vi "ServerRedo.vi"() -> ()   [LabVIEW 2021]
panel:
  in  "stop":bool
  in  "Tamper":cluster{u32, u32}[](array[cluster])
  in  "Alarm":cluster{u32, u32}[](array[cluster])
  in  "Bypass":cluster{u32, u32}[](array[cluster])
  in  "Normal":cluster{u32, u32}[](array[cluster])
  out "Zone 6":bool
  out "Zone 5":bool
  out "Zone 4":bool
  out "Zone 3":bool
  out "Zone 2":bool
  out "Zone 1":bool
  # "Green = Normal\nRed = Alarm\nOrange = Tamper\nBlue = Bypass"
  # "Zone Status Indicators"
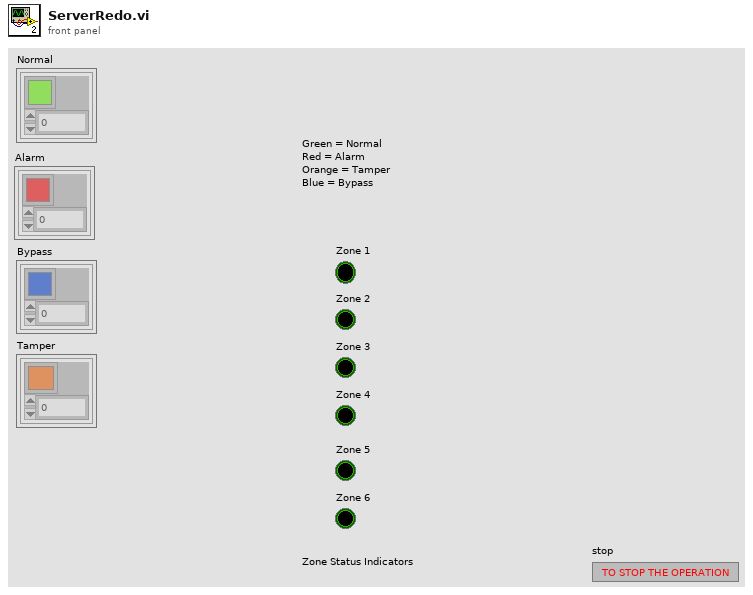
[diagram p1: front panel]
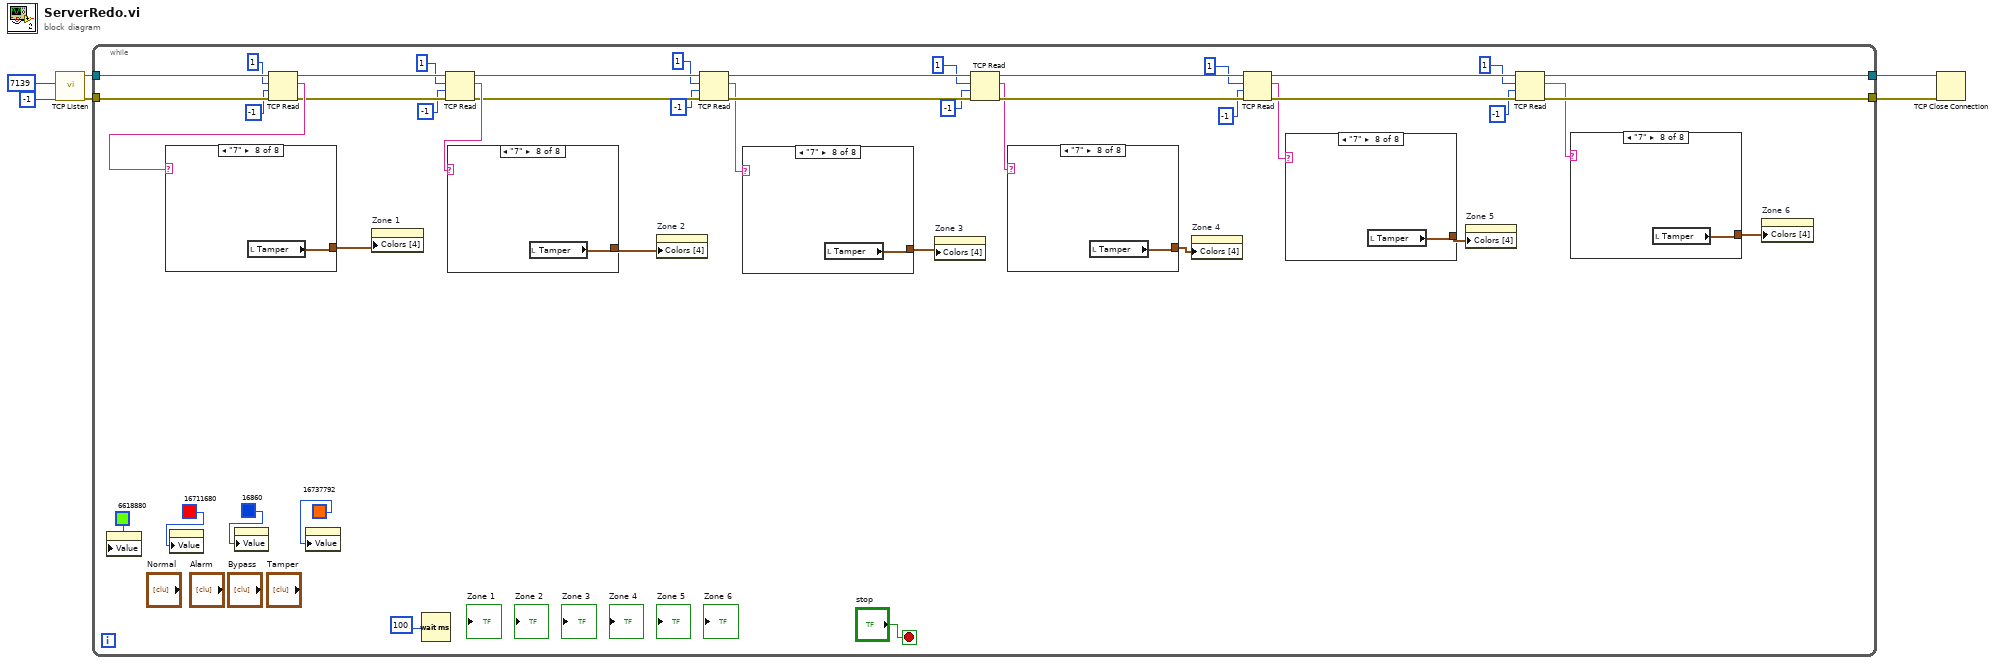
[diagram p0: block diagram]
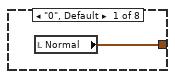
[diagram p2: hidden frame]
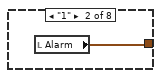
[diagram p3: hidden frame]
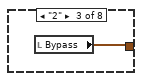
[diagram p4: hidden frame]
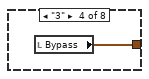
[diagram p5: hidden frame]
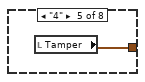
[diagram p6: hidden frame]
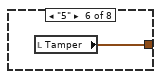
[diagram p7: hidden frame]
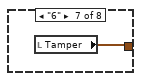
[diagram p8: hidden frame]
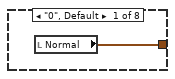
[diagram p9: hidden frame]
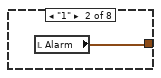
[diagram p10: hidden frame]
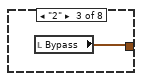
[diagram p11: hidden frame]
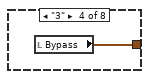
[diagram p12: hidden frame]
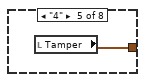
[diagram p13: hidden frame]
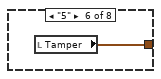
[diagram p14: hidden frame]
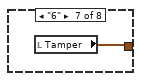
[diagram p15: hidden frame]
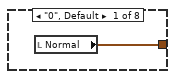
[diagram p16: hidden frame]
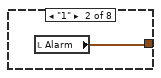
[diagram p17: hidden frame]
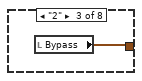
[diagram p18: hidden frame]
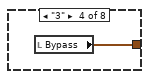
[diagram p19: hidden frame]
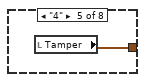
[diagram p20: hidden frame]
diagram:
  n1 = call <vilib>:"TCP Listen.vi"("timeout ms (wait forever: -1)"=-1, "port"=u16 7139) -> ("error out"=w2:errorcluster, "connection ID"=w4:refnum<k5>)  [unwired: 5 in, 3 out]
  n2 = while {
    tunnel: w4 -> [w50]
    tunnel: [w27] -> w3
    tunnel: w2 -> [w49]
    tunnel: [w23] -> w1
    stop <- "stop" stop-if-true
    n3 = property class="ColBox"("Value"=u32 6618880) -> ()  [unwired: 2 in, 2 out]
    n4 = property class="ColBox"("Value"=u32 16711680) -> ()  [unwired: 2 in, 2 out]
    n5 = property class="ColBox"("Value"=u32 16860) -> ()  [unwired: 2 in, 2 out]
    n6 = TCP Read(connection ID=w50, bytes to read=1, error in (no error)=w49, 9:-1 ("timeout ms (25000)")) -> (connection ID out=w38:refnum<k5>, data out=w46:string, error out=w37:errorcluster)  [unwired: 1 in]
    n7 = case shown="\"7\"" w46 {
      tunnel: [w91 w92 w93 w94 w95 w96 w97 w98] -> w45
      frame "0", Default {
        n8 = local read "Normal"() -> (w91:cluster{u32, u32}[])
      }
      frame "1" {
        n9 = local read "Alarm"() -> (w92:cluster{u32, u32}[])
      }
      frame "2" {
        n10 = local read "Bypass"() -> (w93:cluster{u32, u32}[])
      }
      frame "3" {
        n11 = local read "Bypass"() -> (w94:cluster{u32, u32}[])
      }
      frame "4" {
        n12 = local read "Tamper"() -> (w95:cluster{u32, u32}[])
      }
      frame "5" {
        n13 = local read "Tamper"() -> (w96:cluster{u32, u32}[])
      }
      frame "6" {
        n14 = local read "Tamper"() -> (w97:cluster{u32, u32}[])
      }
      frame "7" {
        n15 = local read "Tamper"() -> (w98:cluster{u32, u32}[])
      }
    }
    n16 = property class="ColBox"("Value"=u32 16737792) -> ()  [unwired: 2 in, 2 out]
    n17 = property on="Zone 1" class="Bool (strict)"("Colors [4]"=w45) -> ()  [unwired: 2 in, 2 out]
    n18 = Wait (ms)(milliseconds to wait=100) -> ()  [unwired: 1 out]
    n19 = TCP Read(connection ID=w38, bytes to read=1, error in (no error)=w37, 9:-1 ("timeout ms (25000)")) -> (connection ID out=w32:refnum<k5>, data out=w35:string, error out=w28:errorcluster)  [unwired: 1 in]
    n20 = case shown="\"7\"" w35 {
      tunnel: [w83 w84 w85 w86 w87 w88 w89 w90] -> w36
      frame "0", Default {
        n21 = local read "Normal"() -> (w83:cluster{u32, u32}[])
      }
      frame "1" {
        n22 = local read "Alarm"() -> (w84:cluster{u32, u32}[])
      }
      frame "2" {
        n23 = local read "Bypass"() -> (w85:cluster{u32, u32}[])
      }
      frame "3" {
        n24 = local read "Bypass"() -> (w86:cluster{u32, u32}[])
      }
      frame "4" {
        n25 = local read "Tamper"() -> (w87:cluster{u32, u32}[])
      }
      frame "5" {
        n26 = local read "Tamper"() -> (w88:cluster{u32, u32}[])
      }
      frame "6" {
        n27 = local read "Tamper"() -> (w89:cluster{u32, u32}[])
      }
      frame "7" {
        n28 = local read "Tamper"() -> (w90:cluster{u32, u32}[])
      }
    }
    n29 = property on="Zone 2" class="Bool (strict)"("Colors [4]"=w36) -> ()  [unwired: 2 in, 2 out]
    n30 = TCP Read(connection ID=w32, bytes to read=1, error in (no error)=w28, 9:-1 ("timeout ms (25000)")) -> (connection ID out=w31:refnum<k5>, data out=w13:string, error out=w26:errorcluster)  [unwired: 1 in]
    n31 = case shown="\"7\"" w13 {
      tunnel: [w75 w76 w77 w78 w79 w80 w81 w82] -> w14
      frame "0", Default {
        n32 = local read "Normal"() -> (w75:cluster{u32, u32}[])
      }
      frame "1" {
        n33 = local read "Alarm"() -> (w76:cluster{u32, u32}[])
      }
      frame "2" {
        n34 = local read "Bypass"() -> (w77:cluster{u32, u32}[])
      }
      frame "3" {
        n35 = local read "Bypass"() -> (w78:cluster{u32, u32}[])
      }
      frame "4" {
        n36 = local read "Tamper"() -> (w79:cluster{u32, u32}[])
      }
      frame "5" {
        n37 = local read "Tamper"() -> (w80:cluster{u32, u32}[])
      }
      frame "6" {
        n38 = local read "Tamper"() -> (w81:cluster{u32, u32}[])
      }
      frame "7" {
        n39 = local read "Tamper"() -> (w82:cluster{u32, u32}[])
      }
    }
    n40 = property on="Zone 3" class="Bool (strict)"("Colors [4]"=w14) -> ()  [unwired: 2 in, 2 out]
    n41 = TCP Read(connection ID=w31, bytes to read=1, error in (no error)=w26, 9:-1 ("timeout ms (25000)")) -> (connection ID out=w30:refnum<k5>, data out=w7:string, error out=w25:errorcluster)  [unwired: 1 in]
    n42 = case shown="\"7\"" w7 {
      tunnel: [w67 w68 w69 w70 w71 w72 w73 w74] -> w12
      frame "0", Default {
        n43 = local read "Normal"() -> (w67:cluster{u32, u32}[])
      }
      frame "1" {
        n44 = local read "Alarm"() -> (w68:cluster{u32, u32}[])
      }
      frame "2" {
        n45 = local read "Bypass"() -> (w69:cluster{u32, u32}[])
      }
      frame "3" {
        n46 = local read "Bypass"() -> (w70:cluster{u32, u32}[])
      }
      frame "4" {
        n47 = local read "Tamper"() -> (w71:cluster{u32, u32}[])
      }
      frame "5" {
        n48 = local read "Tamper"() -> (w72:cluster{u32, u32}[])
      }
      frame "6" {
        n49 = local read "Tamper"() -> (w73:cluster{u32, u32}[])
      }
      frame "7" {
        n50 = local read "Tamper"() -> (w74:cluster{u32, u32}[])
      }
    }
    n51 = property on="Zone 4" class="Bool (strict)"("Colors [4]"=w12) -> ()  [unwired: 2 in, 2 out]
    n52 = TCP Read(connection ID=w30, bytes to read=1, error in (no error)=w25, 9:-1 ("timeout ms (25000)")) -> (connection ID out=w29:refnum<k5>, data out=w8:string, error out=w24:errorcluster)  [unwired: 1 in]
    n53 = case shown="\"7\"" w8 {
      tunnel: [w59 w60 w61 w62 w63 w64 w65 w66] -> w11
      frame "0", Default {
        n54 = local read "Normal"() -> (w59:cluster{u32, u32}[])
      }
      frame "1" {
        n55 = local read "Alarm"() -> (w60:cluster{u32, u32}[])
      }
      frame "2" {
        n56 = local read "Bypass"() -> (w61:cluster{u32, u32}[])
      }
      frame "3" {
        n57 = local read "Bypass"() -> (w62:cluster{u32, u32}[])
      }
      frame "4" {
        n58 = local read "Tamper"() -> (w63:cluster{u32, u32}[])
      }
      frame "5" {
        n59 = local read "Tamper"() -> (w64:cluster{u32, u32}[])
      }
      frame "6" {
        n60 = local read "Tamper"() -> (w65:cluster{u32, u32}[])
      }
      frame "7" {
        n61 = local read "Tamper"() -> (w66:cluster{u32, u32}[])
      }
    }
    n62 = property on="Zone 5" class="Bool (strict)"("Colors [4]"=w11) -> ()  [unwired: 2 in, 2 out]
    n63 = TCP Read(connection ID=w29, bytes to read=1, error in (no error)=w24, 9:-1 ("timeout ms (25000)")) -> (connection ID out=w27:refnum<k5>, data out=w9:string, error out=w23:errorcluster)  [unwired: 1 in]
    n64 = case shown="\"7\"" w9 {
      tunnel: [w51 w52 w53 w54 w55 w56 w57 w58] -> w10
      frame "0", Default {
        n65 = local read "Normal"() -> (w51:cluster{u32, u32}[])
      }
      frame "1" {
        n66 = local read "Alarm"() -> (w52:cluster{u32, u32}[])
      }
      frame "2" {
        n67 = local read "Bypass"() -> (w53:cluster{u32, u32}[])
      }
      frame "3" {
        n68 = local read "Bypass"() -> (w54:cluster{u32, u32}[])
      }
      frame "4" {
        n69 = local read "Tamper"() -> (w55:cluster{u32, u32}[])
      }
      frame "5" {
        n70 = local read "Tamper"() -> (w56:cluster{u32, u32}[])
      }
      frame "6" {
        n71 = local read "Tamper"() -> (w57:cluster{u32, u32}[])
      }
      frame "7" {
        n72 = local read "Tamper"() -> (w58:cluster{u32, u32}[])
      }
    }
    n73 = property on="Zone 6" class="Bool (strict)"("Colors [4]"=w10) -> ()  [unwired: 2 in, 2 out]
  }
  n74 = TCP Close Connection(connection ID=w3, error in (no error)=w1) -> ()  [unwired: 1 in, 2 out]
